vi "IMAQ FPGA Camera Link Line Builder.vi"   [LabVIEW 2020]
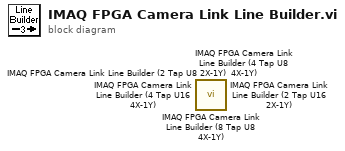
[diagram p0: block diagram]
diagram:
  n1 = call <vilib>:"IMAQ FPGA Camera Link Line Builder (8 Tap U8 4X-1Y).vi"() -> ()  [unwired: 7 in, 5 out]
  n2 = call <vilib>:"IMAQ FPGA Camera Link Line Builder (4 Tap U8 4X-1Y).vi"() -> ()  [unwired: 7 in, 5 out]
  n3 = call <vilib>:"IMAQ FPGA Camera Link Line Builder (4 Tap U16 4X-1Y).vi"() -> ()  [unwired: 7 in, 5 out]
  n4 = call <vilib>:"IMAQ FPGA Camera Link Line Builder (2 Tap U16 2X-1Y).vi"() -> ()  [unwired: 7 in, 5 out]
  n5 = call <vilib>:"IMAQ FPGA Camera Link Line Builder (2 Tap U8 2X-1Y).vi"() -> ()  [unwired: 7 in, 5 out]
